vi "Initialize Font.vi"(11 "error in (no error)":errorcluster) -> (4 "Font OUT":refnum<class "Font Class.lvclass">, 15 "error out":errorcluster)   [LabVIEW 2020, in "Exaprom PDF.lvlib" / "Font Class.lvclass"]
uses:
  <userlib>/labview-PDF-writer-master/LV Class/Fonts Class/Font Class.lvclass
  <userlib>/labview-PDF-writer-master/Controls/Font Controls/Font complete cluster.ctl
  <userlib>/labview-PDF-writer-master/Controls/Font Controls/Font size.ctl
  <userlib>/labview-PDF-writer-master/Controls/Font Controls/Font color.ctl
  <userlib>/labview-PDF-writer-master/Controls/Font Controls/Type and encoding.ctl
  <userlib>/labview-PDF-writer-master/Controls/Text Controls/Unicode/Type and run direction.ctl
  <userlib>/labview-PDF-writer-master/LV Class/Fonts Class/Font Class.lvclass/Font Class.ctl
  <userlib>/labview-PDF-writer-master/Exaprom PDF.lvlib
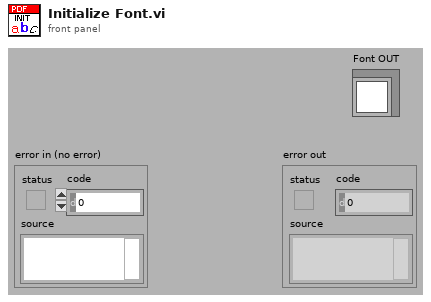
[diagram p1: front panel]
types:
  T1 = typedef "Exaprom PDF.lvlib/Font complete cluster.ctl" = cluster{"Name":string, "Size":T2, "Color":T3, "Style":cluster{"Bold":bool, "Italic":bool, "Underline":bool, "Strikeout":bool}, "Type":T4}
  T2 = typedef "Exaprom PDF.lvlib/Font size.ctl" = sgl
  T3 = typedef "Exaprom PDF.lvlib/Font color.ctl" = u32
  T4 = typedef "Exaprom PDF.lvlib/Type and encoding.ctl" = cluster{"Type&direction":T5, "Embedded":bool, "Encoding":string}
  T5 = typedef "Exaprom PDF.lvlib/Type and run direction.ctl" = enum16{"Select", "ASCII", "UTF-16", "UTF-16 (default)", "UTF-16 (LTR)", "UTF-16 (RTL)"}
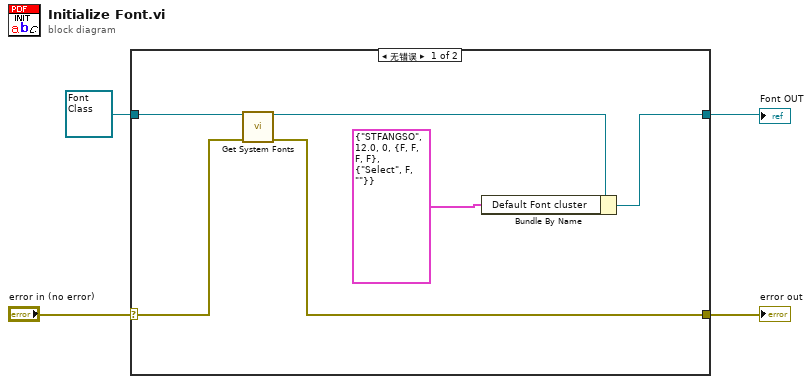
[diagram p0: block diagram]
diagram:
  n1 = case shown="无错误" "error in (no error)" {
    selector: "error in (no error)" -> [w7 w12]
    tunnel: [w6 w12] -> w3
    tunnel: [w10 w11] -> w2
    tunnel: refnum<class "Font Class.lvclass"> refnum ("Font IN") -> [w5 w11]
    frame No Error {
      n2 = call <userlib>:"Get System Fonts.vi"("Font IN"=w5, "error in (no error)"=w7) -> ("Font OUT"=w8:refnum<class "Font Class.lvclass">, "error out"=w6:errorcluster)  [unwired: 12 in]
      n3 = Bundle By Name(cluster=w8, "Default Font cluster"=T1 {"Name"="STFANGSO", "Size"=12.0, "Color"=0, "Style"={"Bold"=FALSE, "Italic"=FALSE, "Underline"=FALSE, "Strikeout"=FALSE}, "Type"={"Type&direction"=enum."Select", "Embedded"=FALSE, "Encoding"=""}}) -> (w10:refnum<class "Font Class.lvclass">)
    }
    frame Error {
    }
  }
  "error out" <- w3
  "Font OUT" <- w2
